vi "SimulBoltek.vi"() -> ()   [LabVIEW 2010]
uses:
  <vilib>/Utility/error.llb/DialogType.ctl
  <vilib>/Instr/_visa.llb/VISA Configure Serial Port (Instr).vi
panel:
  in  "Output rate":sgl(slide) scale=0.5..4.0
  in  "parity":enum16{"None", "Odd", "Even", "Mark", "Space"}(ring)=enum."Odd"
  in  "port number":refnum<visa-resource-name>="COM7"
  in  "+ o -":bool
  in  "data bit":i32=7
  in  "badFormat?":bool
  out "Boolean":bool
  in  "baud rate":u32=2400
  in  "noise?":bool
  in  "constant input?":bool
  in  "go 2":bool
  out "data string 2":string
  out "COM err msg:":string="No Error"
  in  "mV":sgl(slide)=1000.0 scale=0.0..30000.0
  # "E-FieldMill SIMULATOR"
  # "E-Field Mill"
  # "Ver 1.5"
  # "SERIAL COMMUNICATION"
  # "ON - OFF"
  # "FEEDBACK"
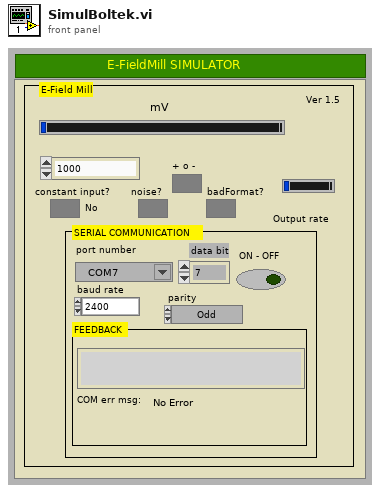
[diagram p1: front panel]
types:
  T1 = typedef "DialogType.ctl" = u16
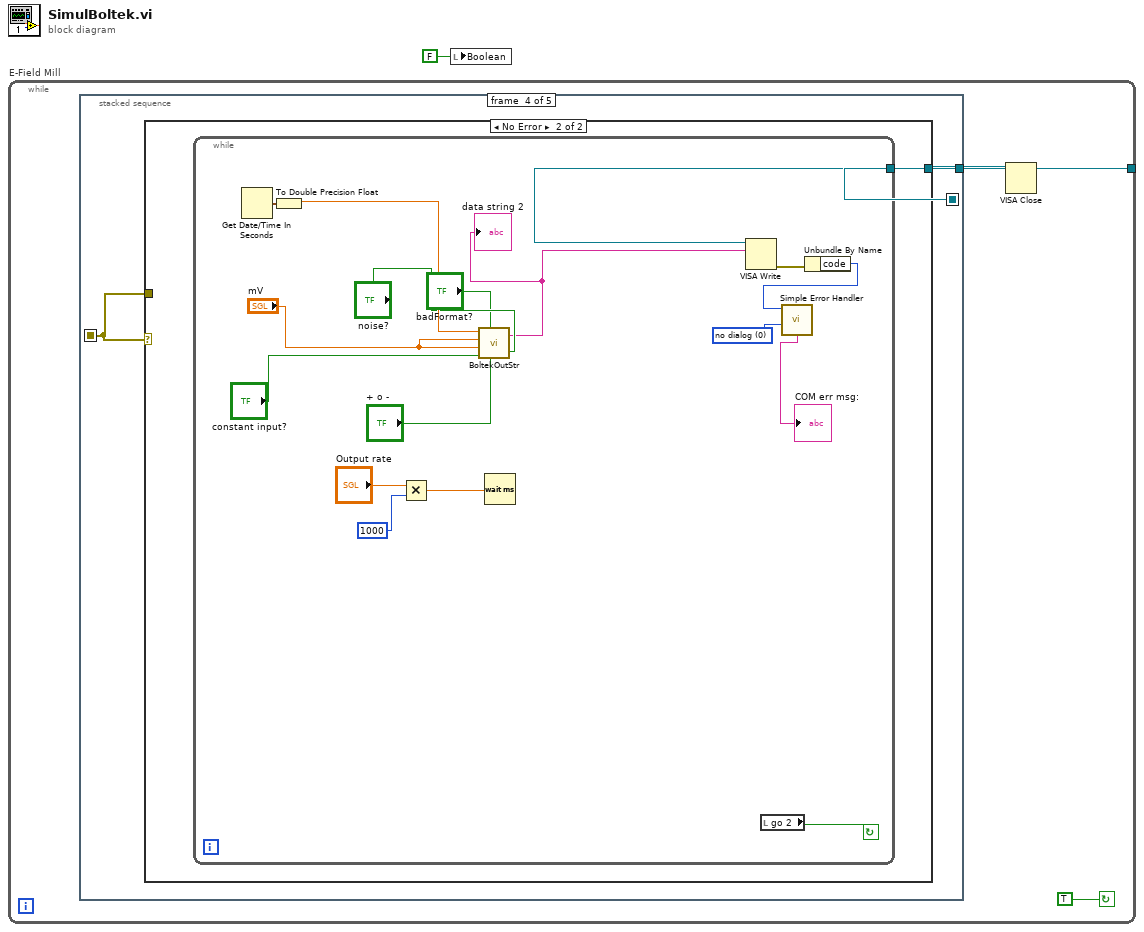
[diagram p0: block diagram]
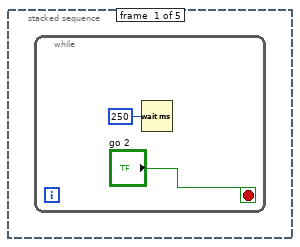
[diagram p2: hidden frame]
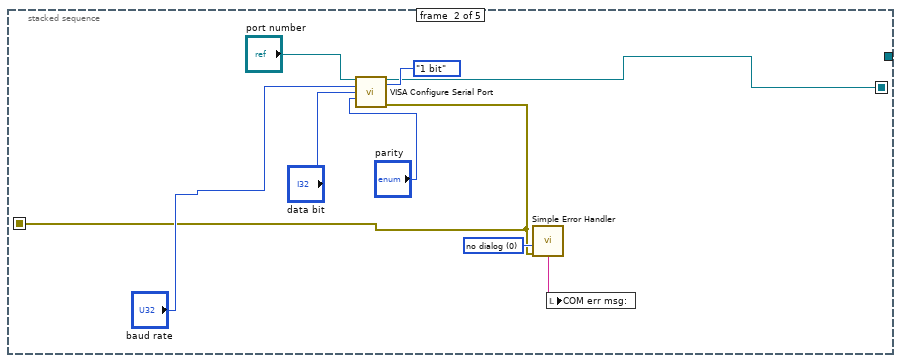
[diagram p3: hidden frame]
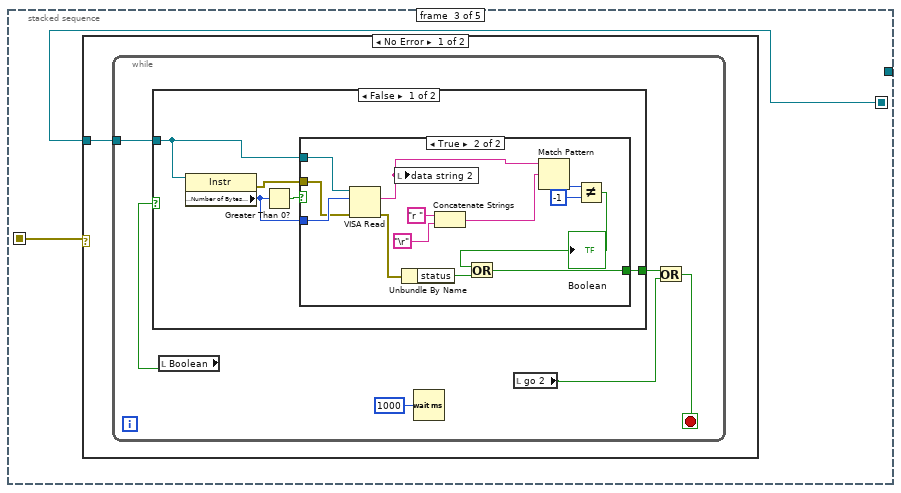
[diagram p4: hidden frame]
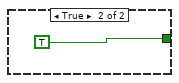
[diagram p6: hidden frame]
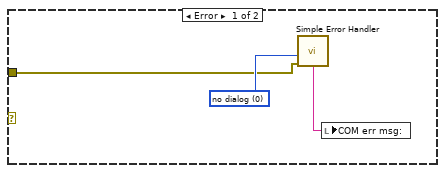
[diagram p8: hidden frame]
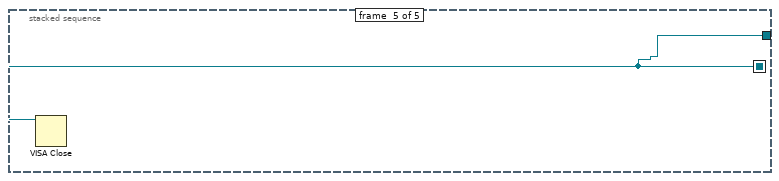
[diagram p9: hidden frame]
diagram:
  n1 = while "E-Field Mill" {
    tunnel: [w3] -> w2
    stop <- TRUE continue-if-true
    n2 = stacked-sequence {
      seq-local: [_ w8 _ _ _] -> [_ _ w17 w45 _]
      seq-local: [_ w11 _ _ _] -> [_ _ w16 w46 w68]
      tunnel: [_ _ _ _ w68] -> w3
      frame #0 {
        n3 = while {
          stop <- "go 2" stop-if-true
          n4 = Wait (ms)(milliseconds to wait=u32 250) -> ()  [unwired: 1 out]
        }
      }
      frame #1 {
        w15 = T1 0 items=["no dialog", "OK message", "continue or stop message", "OK message + warnings", "continue/stop + warnings"] ("type of dialog (OK msg:1)")
        n5 = call-poly "VISA Configure Serial Port"("VISA resource name"="port number", "termination char\n(0xA = '\\n' = LF)"=enum16{"1 bit", "1.5 bits", "2 bits"}."1 bit" ("stop bits"), "baud rate (9600)"="baud rate", "data bits (8)"="data bit", "parity (0:none)"="parity") -> ("VISA resource name out"=w11:refnum<visa-resource-name>, "error out"=w8:errorcluster)  [unwired: 9 in]
        n6 = call <vilib>:"Simple Error Handler.vi"("type of dialog (OK msg:1)"=w15, "error in (no error)"=w8) -> ("message"=w14:string)  [unwired: 3 in, 4 out]
        n7 = local write "COM err msg:"(w14) -> ()
      }
      frame #2 {
        n8 = case shown="No Error" w17 {
          tunnel: w16 -> [w18 _]
          frame No Error {
            n9 = while {
              tunnel: w18 -> [w24]
              stop <- w21 stop-if-true
              n10 = local read "Boolean"() -> (w20:bool)
              n11 = case shown="False" w20 {
                tunnel: w24 -> [w28 _]
                tunnel: [w25 TRUE] -> w22
                frame False {
                  n12 = property class="Instr"(reference=w28) -> (error out=w26:errorcluster, "Serial Settings:Number of Bytes at Serial Port"=w27:u32)  [unwired: 1 in, 1 out]
                  n13 = Greater Than 0?(x=w27) -> (x > 0?=w29:bool)
                  n14 = case shown="True" w29 {
                    selector: w29 -> [w30 _]
                    tunnel: w28 -> [_ w43]
                    tunnel: w27 -> [_ w42]
                    tunnel: w26 -> [_ w41]
                    tunnel: [w30 w32] -> w25
                    frame False {
                    }
                    frame True {
                      n15 = VISA Read(VISA resource name=w43, byte count=w42, error in (no error)=w41) -> (read buffer=w35:string, error out=w38:errorcluster)  [unwired: 2 out]
                      n16 = local write "data string 2"(w35) -> ()
                      n17 = Unbundle By Name(w38) -> ("status"=w37:bool)
                      n18 = Concatenate Strings("r " ("string"), "\r") -> (w36:string)
                      n19 = Match Pattern(string=w35, regular expression=w36) -> (offset past match=w34:i32)  [unwired: 1 in, 3 out]
                      n20 = Not Equal?(x=w34, y=-1) -> (x != y?=w31:bool)
                      "Boolean" <- w31
                      n21 = Or(x=w31, y=w37) -> (x .or. y?=w32:bool)
                    }
                  }
                }
                frame True {
                }
              }
              n22 = Wait (ms)(milliseconds to wait=u32 1000) -> ()  [unwired: 1 out]
              n23 = local read "go 2"() -> (w19:bool)
              n24 = Or(x=w22, y=w19) -> (x .or. y?=w21:bool)
            }
          }
          frame Error {
          }
        }
      }
      frame #3 {
        n25 = case shown="No Error" w45 {
          tunnel: w45 -> [w47 _]
          tunnel: w46 -> [_ w50]
          frame Error {
            w48 = T1 0 items=["no dialog", "OK message", "continue or stop message", "OK message + warnings", "continue/stop + warnings"] ("type of dialog (OK msg:1)")
            n26 = call <vilib>:"Simple Error Handler.vi"("type of dialog (OK msg:1)"=w48, "error in (no error)"=w47) -> ("message"=w49:string)  [unwired: 3 in, 4 out]
            n27 = local write "COM err msg:"(w49) -> ()
          }
          frame No Error {
            n28 = while {
              tunnel: w50 -> [w63]
              stop <- w59 continue-if-true
              w57 = T1 0 items=["no dialog", "OK message", "continue or stop message", "OK message + warnings", "continue/stop + warnings"] ("type of dialog (OK msg:1)")
              n29 = Get Date/Time In Seconds() -> (seconds since 1Jan1904=w66:timestamp)
              n30 = To Double Precision Float(number=w66) -> (double precision float=w67:dbl)
              n31 = Multiply(x="Output rate", y=u32 1000) -> (x*y=w51:sgl)
              n32 = call "BoltekOutStr.vi"("noise?"="noise?", "+ or -"="+ o -", "badFormat?"="badFormat?", "inputs_constant?"="constant input?", "Kv/m Amplitude"="mV", "constant"="mV", "seconds since 1Jan1904"=w67) -> ("String Boltek"=w58:string)
              "data string 2" <- w58
              n33 = Wait (ms)(milliseconds to wait=w51) -> ()  [unwired: 1 out]
              n34 = VISA Write(VISA resource name=w63, write buffer=w58) -> (error out=w65:errorcluster)  [unwired: 1 in, 2 out]
              n35 = local read "go 2"() -> (w59:bool)
              n36 = Unbundle By Name(w65) -> ("code"=w64:i32)
              n37 = call <vilib>:"Simple Error Handler.vi"("error code (no error:0)"=w64, "type of dialog (OK msg:1)"=w57) -> ("message"=→"COM err msg:":string)  [unwired: 3 in, 4 out]
            }
          }
        }
      }
      frame #4 {
        n38 = VISA Close(VISA resource name=w68) -> ()  [unwired: 1 in, 1 out]
      }
    }
  }
  n39 = local write "Boolean"(FALSE ("Boolean")) -> ()
  n40 = VISA Close(VISA resource name=w2) -> ()  [unwired: 1 in, 1 out]
